vi "Clone Template Actor.vi"(8 "error in (no error)":errorcluster, 11 "Destination Directory":path) -> (0 "error out":errorcluster)   [LabVIEW 2018, in "Templates.lvlib"]
uses:
  Templates.lvlib
  Templates/Actor/Actor.lvclass
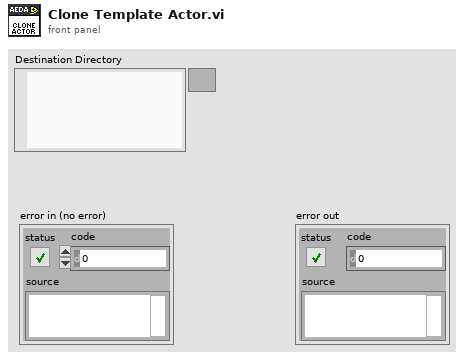
[diagram p1: front panel]
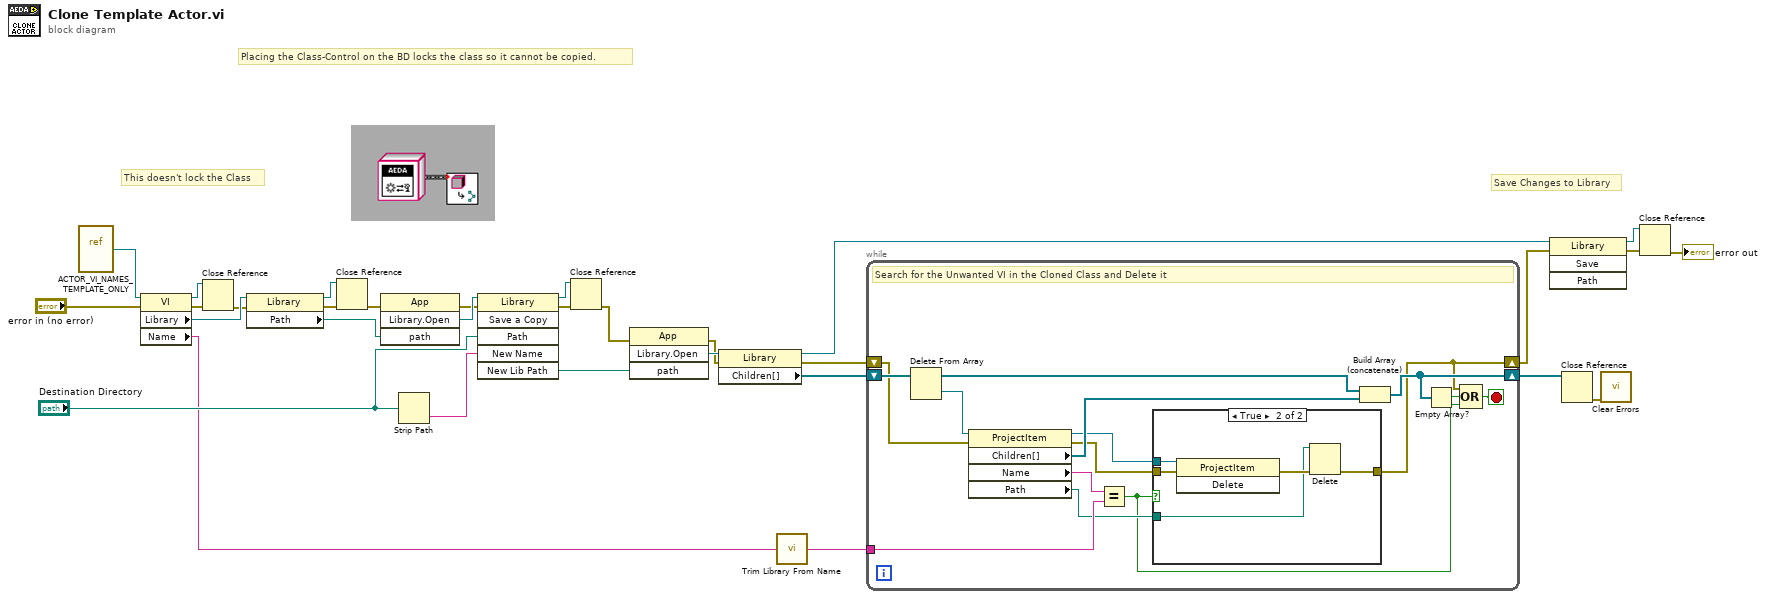
[diagram p0: block diagram]
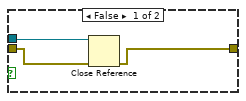
[diagram p2: hidden frame]
diagram:
  # "Save Changes to Library"
  # "This doesn't lock the Class"
  # "Placing the Class-Control on the BD locks the class so it cannot be copied."
  n1 = vi-ref "ACTOR_VI_NAMES_TEMPLATE_ONLY.vi"() -> (w15:refnum<vi>)
  n2 = property class="VI"(reference=w15, error in="error in (no error)") -> (reference out=w13:refnum<vi>, error out=w14:errorcluster, "Library"=w16:refnum<vi>, "Name"=w11:string)
  n3 = Close Reference(reference=w13, error in (no error)=w14) -> (error out=w12:errorcluster)
  n4 = property class="Library"(reference=w16, error in=w12) -> (reference out=w22:refnum<vi>, error out=w23:errorcluster, "Path"=w25:path)
  n5 = Close Reference(reference=w22, error in (no error)=w23) -> (error out=w21:errorcluster)
  n6 = invoke class="App" method="Library.Open"(error in=w21, "path"=w25) -> (error out=w28:errorcluster, "Open Library"=w31:refnum<vi>)  [unwired: 2 in, 2 out]
  n7 = Strip Path(path="Destination Directory") -> (name=w29:string)  [unwired: 1 out]
  n8 = invoke class="Library" method="Save a Copy"(reference=w31, error in=w28, "Path"="Destination Directory", "New Name"=w29) -> (reference out=w27:refnum<vi>, error out=w26:errorcluster, "New Lib Path"=w10:path)  [unwired: 2 in, 3 out]
  n9 = Close Reference(reference=w27, error in (no error)=w26) -> (error out=w20:errorcluster)
  n10 = invoke class="App" method="Library.Open"(error in=w20, "path"=w10) -> (error out=w18:errorcluster, "Open Library"=w19:refnum<vi>)  [unwired: 2 in, 2 out]
  n11 = property class="Library"(reference=w19, error in=w18) -> (reference out=w5:refnum<vi>, error out=w6:errorcluster, "Children[]"=w17:refnum<vi>[])
  n12 = call "Trim Library From Name.vi"("Name in"=w11) -> ("Name out"=w9:string)
  n13 = while {
    shift-right: [w42] -> w8
    shift-left: w17 -> [w46]
    shift-right: [w32] -> w4
    shift-left: w6 -> [w43]
    tunnel: w9 -> [w39]
    stop <- w33 stop-if-true
    # "Search for the Unwanted VI in the Cloned Class and Delete it"
    n14 = Delete From Array(array=w46) -> (deleted portion=w41:refnum<vi>, array with subset deleted=w45:refnum<vi>[])  [unwired: 2 in]
    n15 = property class="ProjectItem"(reference=w41, error in=w43) -> (reference out=w38:refnum<vi>, error out=w36:errorcluster, "Children[]"=w44:refnum<vi>[], "Name"=w40:string, "Path"=w37:path)
    n16 = Equal?(x=w40, y=w39) -> (x = y?=w34:bool)
    n17 = case shown="True" w34 {
      tunnel: w38 -> [w49 w54]
      tunnel: w37 -> [_ w51]
      tunnel: w36 -> [w48 w53]
      tunnel: [w47 w50] -> w32
      frame False {
        n18 = Close Reference(reference=w49, error in (no error)=w48) -> (error out=w47:errorcluster)
      }
      frame True {
        n19 = invoke class="ProjectItem" method="Delete"(reference=w54, error in=w53) -> (error out=w52:errorcluster)  [unwired: 1 in, 2 out]
        n20 = Delete(path (use dialog)=w51, error in=w52) -> (error out=w50:errorcluster)  [unwired: 3 in, 2 out]
      }
    }
    n21 = Build Array (concatenate)(w45, w44) -> (w42:refnum<vi>[])
    n22 = Empty Array?(array=w42) -> (empty?=w35:bool)
    n23 = Compound Arithmetic op=OR(w32, w35, w34) -> (w33:bool)
  }
  n24 = invoke class="Library" method="Save"(reference=w5, error in=w4) -> (reference out=w2:refnum<vi>, error out=w3:errorcluster)  [unwired: 2 in, 2 out]
  n25 = Close Reference(reference=w8) -> (error out=w7:errorcluster)  [unwired: 1 in]
  n26 = call <vilib>:"Clear Errors.vi"("error in (no error)"=w7) -> ()  [unwired: 5 in, 2 out]
  n27 = Close Reference(reference=w2, error in (no error)=w3) -> (error out=→"error out":errorcluster)
